vi "Signal.FG.vi"(7 "Action":T1, 8 "error in (no error)":errorcluster, 10 "Signal Parameters":T2 {"Byte Order" items=["Little Endian", "Big Endian"]; "Data Type" items=["Signed", "Unsigned", "IEEE Float"]}, 11 "Device Item Ref in":T3 format="%.0x") -> (0 "error out":errorcluster, 2 "Signal Parameters":T2 {"Byte Order" items=["Little Endian", "Big Endian"]; "Data Type" items=["Signed", "Unsigned", "IEEE Float"]}, 3 "Device Item Ref out":T3=18446744073709551615 format="%.0x")   [LabVIEW 2024, in "Diagnostics Addon System Explorer.lvlib"]
uses:
  Diagnostics Addon System Explorer.lvlib
  <vilib>/NI VeriStand/Custom Device API/Custom Device Item Ref.ctl
  Addon Shared/Types/Signal.ctl
  Types/FG.Action.ctl
  Addon Shared/SubVIs/Constants.vi
  <vilib>/NI/NI VeriStand Advanced SysDef API/_SubVIs/SysDef.Property.Set.U32.vi
  <vilib>/NI/NI VeriStand Advanced SysDef API/_SubVIs/SysDef.Property.Set.DBL.vi
  <vilib>/NI/NI VeriStand Advanced SysDef API/_SubVIs/SysDef.Property.Set.String.vi
  <vilib>/NI VeriStand/Custom Device API/Get Item Property (U32).vi
  <vilib>/NI VeriStand/Custom Device API/Get Item Property (Double).vi
  <vilib>/NI VeriStand/Custom Device API/Get Item Property (String).vi
  Addon Shared/Diagnostics Addon Shared.lvlib
  <vilib>/NI VeriStand/Custom Device API/Custom Device API.lvlib
  <vilib>/NI/NI VeriStand Advanced SysDef API/SysDef API/Advanced System Definition.lvlib
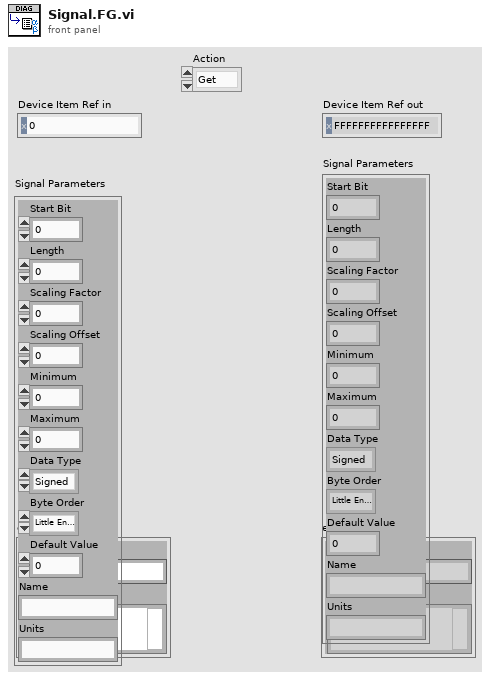
[diagram p1: front panel]
types:
  T1 = typedef "Diagnostics Addon System Explorer.lvlib/FG.Action.ctl" = enum16{"Get", "Set"}
  T2 = typedef "Diagnostics Addon Shared.lvlib/Signal.ctl" = cluster{"Start Bit":u32, "Length":u32, "Scaling Factor":dbl, "Scaling Offset":dbl, "Minimum":dbl, "Maximum":dbl, "Data Type":u32, "Byte Order":u32, "Default Value":dbl, "Name":string, "Units":string}
  T3 = typedef "Custom Device API.lvlib/Custom Device Item Ref.ctl" = u64
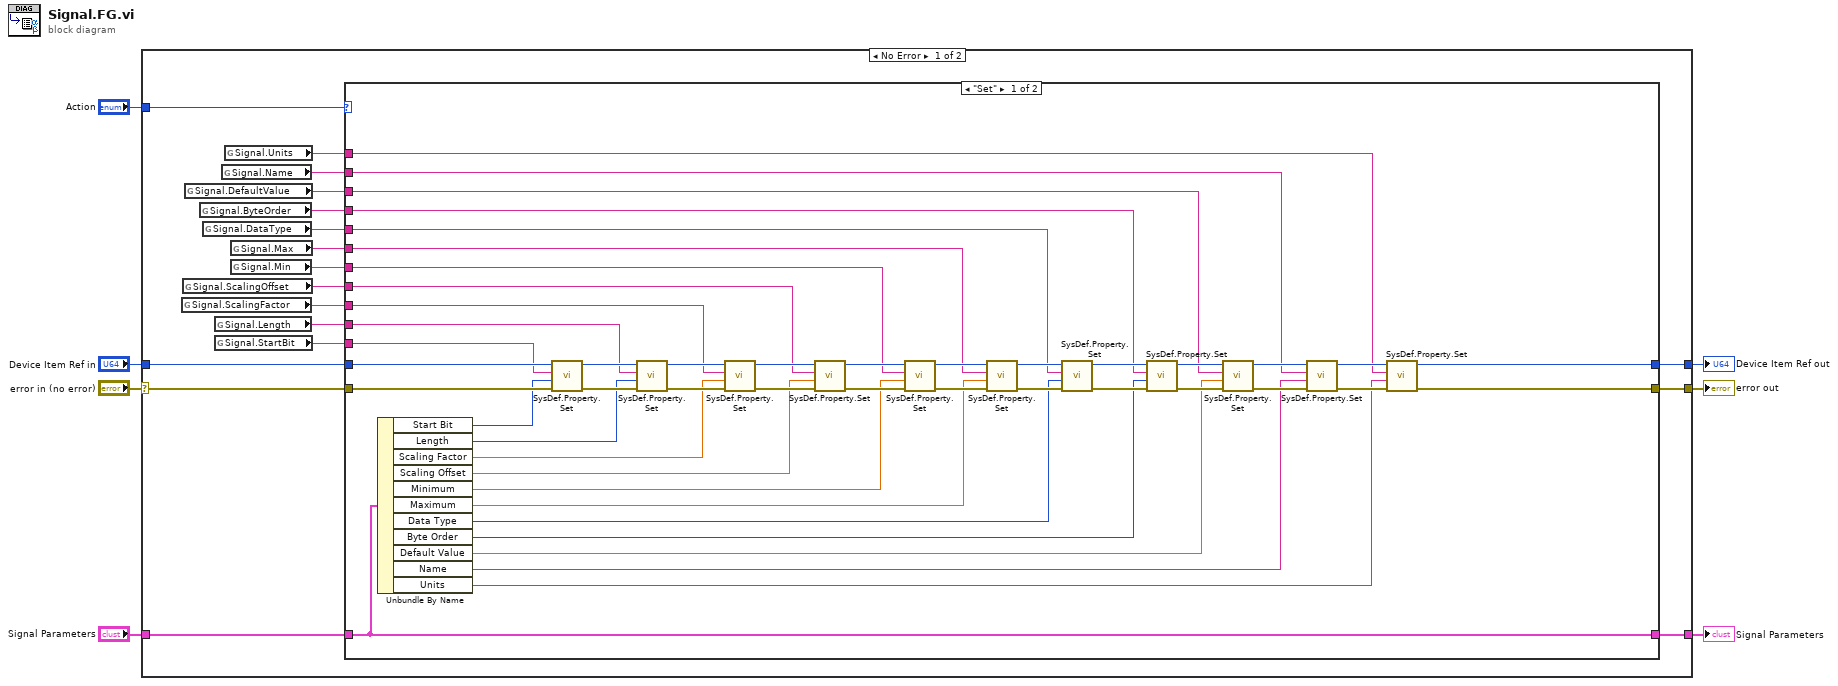
[diagram p0: block diagram]
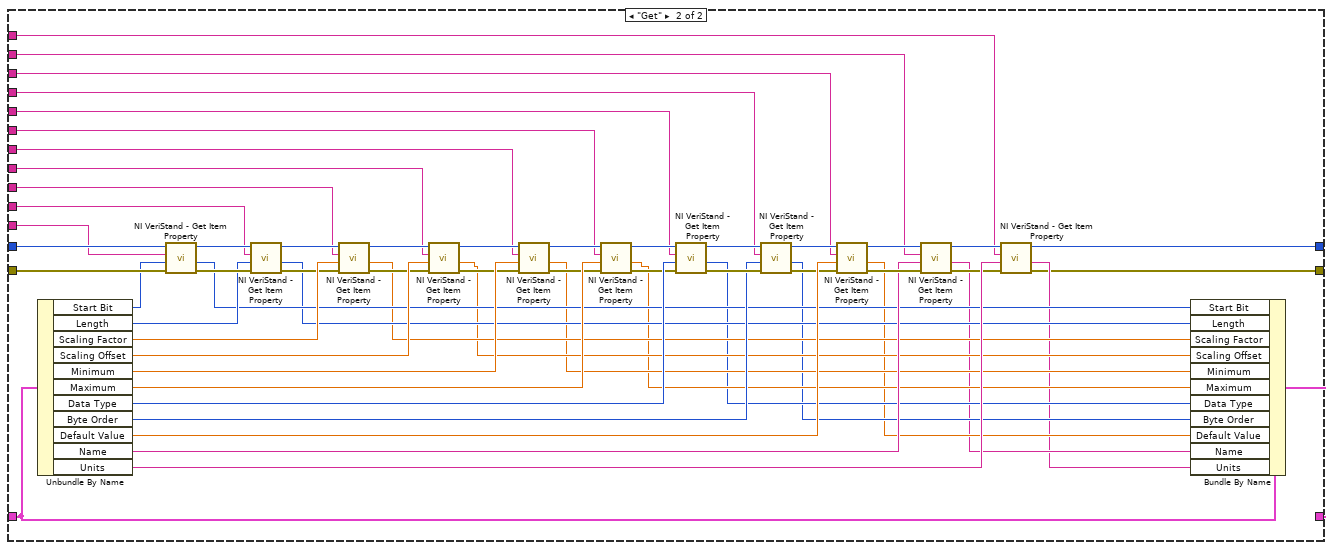
[diagram p2: hidden frame]
diagram:
  n1 = case shown="No Error" "error in (no error)" {
    selector: "error in (no error)" -> [w25 w132]
    tunnel: "Device Item Ref in" -> [w24 w133]
    tunnel: [w23 w133] -> w4
    tunnel: [w22 w132] -> w5
    tunnel: [w21 _] -> w3
    tunnel: "Signal Parameters" -> [w20 _]
    tunnel: "Action" -> [w19 _]
    frame No Error {
      n2 = global read "Constants.vi" "Signal.ScalingFactor"() -> (w16:string)
      n3 = global read "Constants.vi" "Signal.ScalingOffset"() -> (w15:string)
      n4 = global read "Constants.vi" "Signal.DefaultValue"() -> (w10:string)
      n5 = global read "Constants.vi" "Signal.ByteOrder"() -> (w11:string)
      n6 = global read "Constants.vi" "Signal.DataType"() -> (w12:string)
      n7 = global read "Constants.vi" "Signal.Length"() -> (w17:string)
      n8 = global read "Constants.vi" "Signal.StartBit"() -> (w18:string)
      n9 = global read "Constants.vi" "Signal.Name"() -> (w9:string)
      n10 = global read "Constants.vi" "Signal.Units"() -> (w8:string)
      n11 = global read "Constants.vi" "Signal.Max"() -> (w13:string)
      n12 = global read "Constants.vi" "Signal.Min"() -> (w14:string)
      n13 = case shown="\"Set\"" w19 {
        tunnel: w25 -> [w61 w131]
        tunnel: w24 -> [w60 w130]
        tunnel: [w26 w73] -> w23
        tunnel: [w27 w74] -> w22
        tunnel: [w62 w75] -> w21
        tunnel: w20 -> [w62 w87]
        tunnel: w18 -> [w29 w99]
        tunnel: w17 -> [w30 w98]
        tunnel: w16 -> [w31 w97]
        tunnel: w15 -> [w32 w96]
        tunnel: w14 -> [w33 w95]
        tunnel: w13 -> [w34 w94]
        tunnel: w12 -> [w35 w93]
        tunnel: w11 -> [w36 w92]
        tunnel: w10 -> [w37 w91]
        tunnel: w9 -> [w38 w89]
        tunnel: w8 -> [w39 w88]
        frame "Set" {
          n14 = Unbundle By Name(w62) -> ("Start Bit"=w49:u32, "Length"=w48:u32, "Scaling Factor"=w47:dbl, "Scaling Offset"=w46:dbl, "Minimum"=w45:dbl, "Maximum"=w44:dbl, "Data Type"=w43:u32, "Byte Order"=w42:u32, "Default Value"=w41:dbl, "Name"=w28:string, "Units"=w40:string)
          n15 = call-poly <vilib>:"SysDef.Property.Set.vi"("error in (no error)"=w61, "Value"=w49, "Property Name"=w29, "nodeID"=w60) -> ("error out"=w72:errorcluster, "nodeID out"=w59:u64)  [unwired: 6 in]
          n16 = call-poly <vilib>:"SysDef.Property.Set.vi"("error in (no error)"=w72, "Value"=w48, "Property Name"=w30, "nodeID"=w59) -> ("error out"=w70:errorcluster, "nodeID out"=w58:u64)  [unwired: 6 in]
          n17 = call-poly <vilib>:"SysDef.Property.Set.vi"("error in (no error)"=w70, "Value"=w47, "Property Name"=w31, "nodeID"=w58) -> ("error out"=w69:errorcluster, "nodeID out"=w57:u64)  [unwired: 6 in]
          n18 = call-poly <vilib>:"SysDef.Property.Set.vi"("error in (no error)"=w69, "Value"=w46, "Property Name"=w32, "nodeID"=w57) -> ("error out"=w68:errorcluster, "nodeID out"=w56:u64)  [unwired: 6 in]
          n19 = call-poly <vilib>:"SysDef.Property.Set.vi"("error in (no error)"=w68, "Value"=w45, "Property Name"=w33, "nodeID"=w56) -> ("error out"=w67:errorcluster, "nodeID out"=w55:u64)  [unwired: 6 in]
          n20 = call-poly <vilib>:"SysDef.Property.Set.vi"("error in (no error)"=w67, "Value"=w44, "Property Name"=w34, "nodeID"=w55) -> ("error out"=w66:errorcluster, "nodeID out"=w54:u64)  [unwired: 6 in]
          n21 = call-poly <vilib>:"SysDef.Property.Set.vi"("error in (no error)"=w66, "Value"=w43, "Property Name"=w35, "nodeID"=w54) -> ("error out"=w71:errorcluster, "nodeID out"=w53:u64)  [unwired: 6 in]
          n22 = call-poly <vilib>:"SysDef.Property.Set.vi"("error in (no error)"=w71, "Value"=w42, "Property Name"=w36, "nodeID"=w53) -> ("error out"=w65:errorcluster, "nodeID out"=w52:u64)  [unwired: 6 in]
          n23 = call-poly <vilib>:"SysDef.Property.Set.vi"("error in (no error)"=w65, "Value"=w41, "Property Name"=w37, "nodeID"=w52) -> ("error out"=w64:errorcluster, "nodeID out"=w51:u64)  [unwired: 6 in]
          n24 = call-poly <vilib>:"SysDef.Property.Set.vi"("error in (no error)"=w64, "Value"=w28, "Property Name"=w38, "nodeID"=w51) -> ("error out"=w63:errorcluster, "nodeID out"=w50:u64)  [unwired: 6 in]
          n25 = call-poly <vilib>:"SysDef.Property.Set.vi"("error in (no error)"=w63, "Value"=w40, "Property Name"=w39, "nodeID"=w50) -> ("error out"=w27:errorcluster, "nodeID out"=w26:u64)  [unwired: 6 in]
        }
        frame "Get" {
          n26 = Unbundle By Name(w87) -> ("Start Bit"=w129:u32, "Length"=w116:u32, "Scaling Factor"=w115:dbl, "Scaling Offset"=w114:dbl, "Minimum"=w113:dbl, "Maximum"=w112:dbl, "Data Type"=w111:u32, "Byte Order"=w110:u32, "Default Value"=w109:dbl, "Name"=w90:string, "Units"=w108:string)
          n27 = call-poly <vilib>:"NI VeriStand - Get Item Property.vi"("error in (no error)"=w131, "Default Value"=w129, "Property Name"=w99, "Item Ref in"=w130) -> ("error out"=w127:errorcluster, "Value"=w86:u32, "Item Ref out"=w128:T3)  [unwired: 4 in, 1 out]
          n28 = call-poly <vilib>:"NI VeriStand - Get Item Property.vi"("error in (no error)"=w127, "Default Value"=w116, "Property Name"=w98, "Item Ref in"=w128) -> ("error out"=w107:errorcluster, "Value"=w85:u32, "Item Ref out"=w126:T3)  [unwired: 4 in, 1 out]
          n29 = call-poly <vilib>:"NI VeriStand - Get Item Property.vi"("error in (no error)"=w107, "Default Value"=w115, "Property Name"=w97, "Item Ref in"=w126) -> ("error out"=w106:errorcluster, "Value"=w84:dbl, "Item Ref out"=w125:T3)  [unwired: 4 in, 1 out]
          n30 = call-poly <vilib>:"NI VeriStand - Get Item Property.vi"("error in (no error)"=w106, "Default Value"=w114, "Property Name"=w96, "Item Ref in"=w125) -> ("error out"=w105:errorcluster, "Value"=w83:dbl, "Item Ref out"=w124:T3)  [unwired: 4 in, 1 out]
          n31 = call-poly <vilib>:"NI VeriStand - Get Item Property.vi"("error in (no error)"=w105, "Default Value"=w113, "Property Name"=w95, "Item Ref in"=w124) -> ("error out"=w104:errorcluster, "Value"=w82:dbl, "Item Ref out"=w123:T3)  [unwired: 4 in, 1 out]
          n32 = call-poly <vilib>:"NI VeriStand - Get Item Property.vi"("error in (no error)"=w104, "Default Value"=w112, "Property Name"=w94, "Item Ref in"=w123) -> ("error out"=w103:errorcluster, "Value"=w81:dbl, "Item Ref out"=w121:T3)  [unwired: 4 in, 1 out]
          n33 = call-poly <vilib>:"NI VeriStand - Get Item Property.vi"("error in (no error)"=w103, "Default Value"=w111, "Property Name"=w93, "Item Ref in"=w121) -> ("error out"=w122:errorcluster, "Value"=w80:u32, "Item Ref out"=w120:T3)  [unwired: 4 in, 1 out]
          n34 = call-poly <vilib>:"NI VeriStand - Get Item Property.vi"("error in (no error)"=w122, "Default Value"=w110, "Property Name"=w92, "Item Ref in"=w120) -> ("error out"=w102:errorcluster, "Value"=w79:u32, "Item Ref out"=w119:T3)  [unwired: 4 in, 1 out]
          n35 = call-poly <vilib>:"NI VeriStand - Get Item Property.vi"("error in (no error)"=w102, "Default Value"=w109, "Property Name"=w91, "Item Ref in"=w119) -> ("error out"=w101:errorcluster, "Value"=w78:dbl, "Item Ref out"=w118:T3)  [unwired: 4 in, 1 out]
          n36 = call-poly <vilib>:"NI VeriStand - Get Item Property.vi"("error in (no error)"=w101, "Default Value"=w90, "Property Name"=w89, "Item Ref in"=w118) -> ("error out"=w100:errorcluster, "Value"=w77:string, "Item Ref out"=w117:T3)  [unwired: 4 in, 1 out]
          n37 = call-poly <vilib>:"NI VeriStand - Get Item Property.vi"("error in (no error)"=w100, "Default Value"=w108, "Property Name"=w88, "Item Ref in"=w117) -> ("error out"=w74:errorcluster, "Value"=w76:string, "Item Ref out"=w73:T3)  [unwired: 4 in, 1 out]
          n38 = Bundle By Name(cluster=w87, "Start Bit"=w86, "Length"=w85, "Scaling Factor"=w84, "Scaling Offset"=w83, "Minimum"=w82, "Maximum"=w81, "Data Type"=w80, "Byte Order"=w79, "Default Value"=w78, "Name"=w77, "Units"=w76) -> (w75:T2)
        }
      }
    }
    frame Error {
    }
  }
  "error out" <- w5
  "Device Item Ref out" <- w4
  "Signal Parameters" <- w3
